vi "Digitizer_Mode_Close.vi"(8 "error in":errorcluster, 11 "Channel Parameters In":T1) -> (0 "error out":errorcluster, 1 "Waveforms Out (Empty)":T2(array[cluster]), 3 "Channel Parameters Reset":T3)   [LabVIEW 2010]
uses:
  Typedef-Channel Parameters.ctl
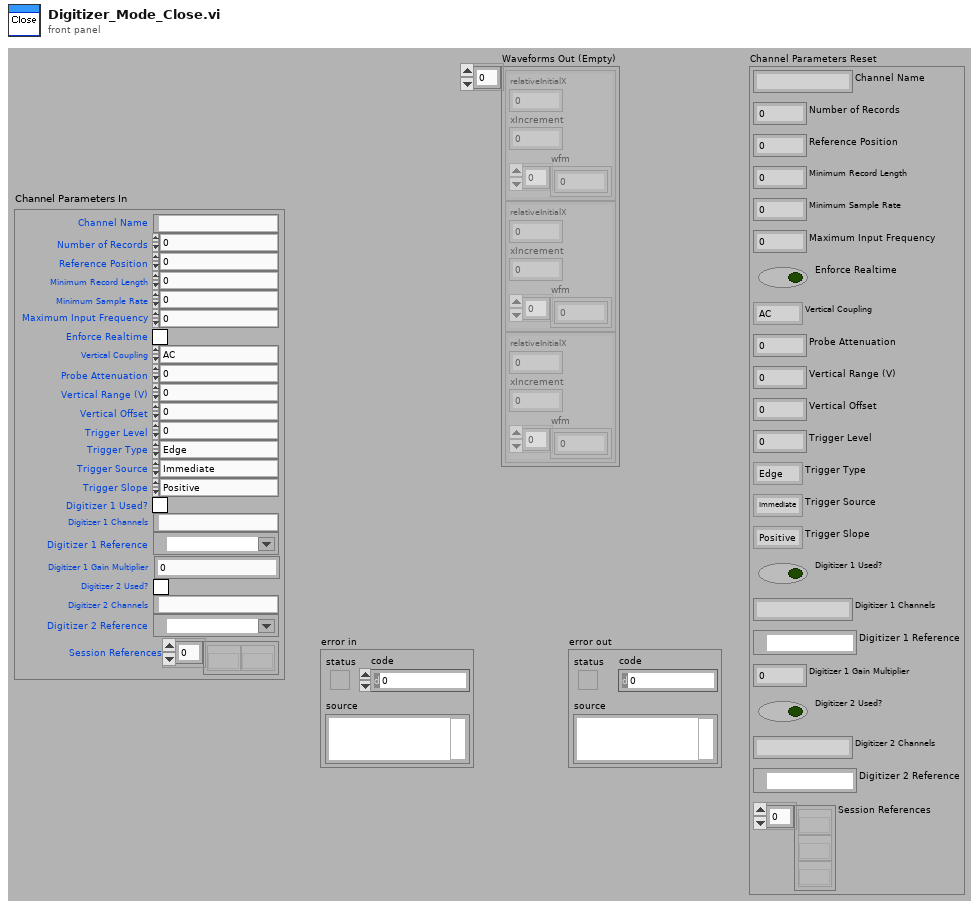
[diagram p1: front panel]
types:
  T1 = typedef "Typedef-Channel Parameters.ctl" = cluster{"Channel Name":string, "Number of Records":i32, "Reference Position":dbl, "Minimum Record Length":i32, "Minimum Sample Rate":dbl, "Maximum Input Frequency":dbl, "Enforce Realtime":bool, "Vertical Coupling":enum16{"AC", "DC", "Ground"}, "Probe Attenuation":dbl, "Vertical Range (V)":dbl, "Vertical Offset":dbl, "Trigger Level":dbl, "Trigger Type":enum16{"Edge", "Digital", "Immediate"}, "Trigger Source":enum16{"Immediate", "Channel 0", "Channel 1", "Channel 2", "Channel 3", "Channel 4", "Channel 5", "Channel 6", "Channel 7", "Extermal TRIG", "Software Trigger", "RTSI 0", "RTSI 1", "RTSI 2", "RTSI 3", "RTSI 4", "RTSI 5", "RTSI 6", "PF 0", "PF 1", "PF 2", "PXI Star Trigger"}, "Trigger Slope":enum16{"Positive", "Negative"}, "Digitizer 1 Used?":bool, "Digitizer 1 Channels":string, "Digitizer 1 Reference":refnum<k15>, "Digitizer 1 Gain Multiplier":dbl, "Digitizer 2 Used?":bool, "Digitizer 2 Channels":string, "Digitizer 2 Reference":refnum<k15>, "Session References":refnum<k20>[]}
  T2 = cluster{"relativeInitialX":dbl, "xIncrement":dbl, "wfm":dbl[]}[]
  T3 = cluster{"Channel Name":string, "Number of Records":i32, "Reference Position":dbl, "Minimum Record Length":i32, "Minimum Sample Rate":dbl, "Maximum Input Frequency":dbl, "Enforce Realtime":bool, "Vertical Coupling":enum16{"AC", "DC", "Ground"}, "Probe Attenuation":dbl, "Vertical Range (V)":dbl, "Vertical Offset":dbl, "Trigger Level":dbl, "Trigger Type":enum16{"Edge", "Digital", "Immediate"}, "Trigger Source":enum16{"Immediate", "Channel 0", "Channel 1", "Channel 2", "Channel 3", "Channel 4", "Channel 5", "Channel 6", "Channel 7", "Extermal TRIG", "Software Trigger", "RTSI 0", "RTSI 1", "RTSI 2", "RTSI 3", "RTSI 4", "RTSI 5", "RTSI 6", "PF 0", "PF 1", "PF 2", "PXI Star Trigger"}, "Trigger Slope":enum16{"Positive", "Negative"}, "Digitizer 1 Used?":bool, "Digitizer 1 Channels":string, "Digitizer 1 Reference":refnum<k15>, "Digitizer 1 Gain Multiplier":dbl, "Digitizer 2 Used?":bool, "Digitizer 2 Channels":string, "Digitizer 2 Reference":refnum<k15>, "Session References":refnum<k20>[]}
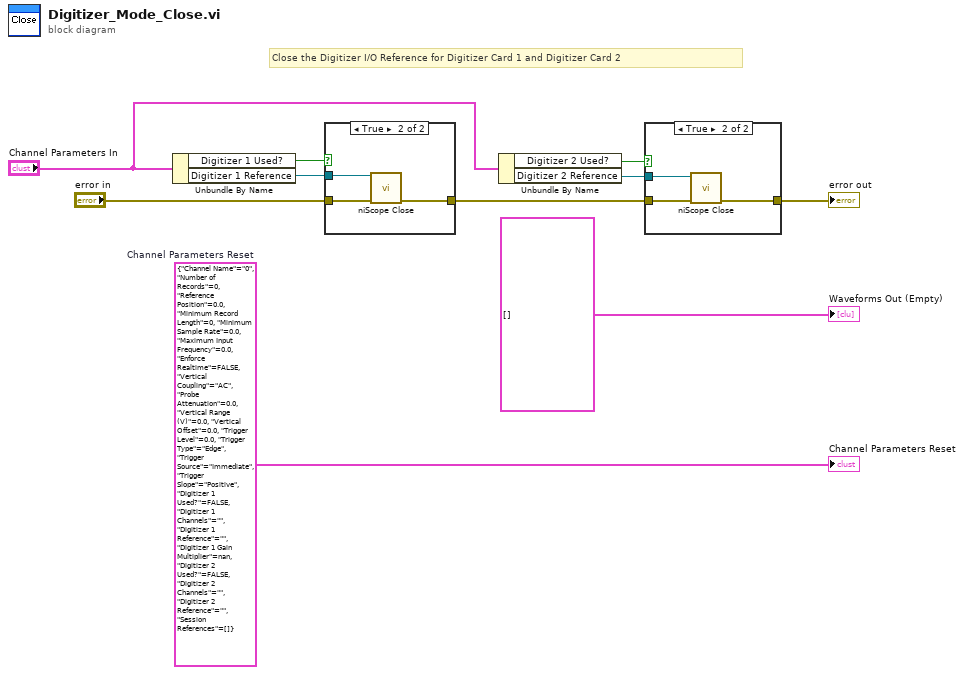
[diagram p0: block diagram]
diagram:
  w1 = T3 {"Channel Name"="0", "Number of Records"=0, "Reference Position"=0.0, "Minimum Record Length"=0, "Minimum Sample Rate"=0.0, "Maximum Input Frequency"=0.0, "Enforce Realtime"=FALSE, "Vertical Coupling"=enum."AC", "Probe Attenuation"=0.0, "Vertical Range (V)"=0.0, "Vertical Offset"=0.0, "Trigger Level"=0.0, "Trigger Type"=enum."Edge", "Trigger Source"=enum."Immediate", "Trigger Slope"=enum."Positive", "Digitizer 1 Used?"=FALSE, "Digitizer 1 Channels"="", "Digitizer 1 Reference"="", "Digitizer 1 Gain Multiplier"=nan, "Digitizer 2 Used?"=FALSE, "Digitizer 2 Channels"="", "Digitizer 2 Reference"="", "Session References"=[]}  # Channel Parameters Reset
  # "Close the Digitizer I/O Reference for Digitizer Card 1 and Digitizer Card 2"
  n1 = Unbundle By Name("Channel Parameters In") -> ("Digitizer 1 Used?"=w4:bool, "Digitizer 1 Reference"=w5:refnum<k15>)
  n2 = case shown="True" w4 {
    tunnel: "error in" -> [w11 w13]
    tunnel: w5 -> [_ w12]
    tunnel: [w11 w14] -> w2
    frame False {
    }
    frame True {
      n3 = call <instrlib>:"niScope Close.vi"("instrument handle"=w12, "error in"=w13) -> ("error out"=w14:errorcluster)  [unwired: 13 in]
    }
  }
  n4 = Unbundle By Name("Channel Parameters In") -> ("Digitizer 2 Used?"=w7:bool, "Digitizer 2 Reference"=w8:refnum<k15>)
  n5 = case shown="True" w7 {
    tunnel: w2 -> [w15 w17]
    tunnel: w8 -> [_ w16]
    tunnel: [w15 w18] -> w3
    frame False {
    }
    frame True {
      n6 = call <instrlib>:"niScope Close.vi"("instrument handle"=w16, "error in"=w17) -> ("error out"=w18:errorcluster)  [unwired: 13 in]
    }
  }
  "error out" <- w3
  "Channel Parameters Reset" <- w1
  "Waveforms Out (Empty)" <- T2 []
